vi "SpecAn_AMPM_ACP_TxP.vi"() -> ()   [LabVIEW 2016]
doc: "This example illustrates how to use the RFmx SpecAn and LTE personalities together with the RFSG drivers to perform ACP and EVM measurements with or without digital predistortion (DPD) of the waveform input to the DUT. \n\nDPD is a technique to optimize the operating point of power amplifiers and other non-linear RFIC devices. Power amplifiers are much more efficient if they operate near compression. However, compressing signal amplitudes can significantly deteriorate the amplified signal's quality both, in-band (e.g., EVM increases due to non-linear distortion of the signal's I/Q constellation) and out-of-band (e.g., ACP or SEM test fails due to spectral regrowth). With DPD, the original waveform is first pre-distorted in a way that matches the non-linear effects of the RFIC device before being fed through the device. The resulting output is a much cleaner amplified and/or filtered version of the original waveform. \n\nDifferent DPD models can be used to trade off performance with computational ease, with the Lookup-Table (LUT) model the simplest and the Generalized Memory Polynomial Model (GMP) the most complex. With a LUT, the DPD algorithm achieves gain and phase linearization on average. If you want to correct for memory effects - i.e., an output sample not only depends on the current input but also previous input samples; you will notice that a specific input power value translates into a range of gain and phase values - you would use one of the memory polynomial models. For these models, several parameters such as polynomial order and memory depth are available to fine-tune the model to the DUT behavior."
uses:
  Source/SG/Typedefs/LO Configruation.ctl
  <instrlib>/niRFSG/niRFSG.llb/niRFSG Exported Signal Destinations.ctl
  Source/SG/Typedefs/Instrument Configuration.ctl
  <instrlib>/niRFSG/niRFSG.llb/niRFSG Ref Clock Sources.ctl
  Source/SA/RFmxSpecAn/Typedefs/AMPM Configuration.ctl
  Source/SA/RFmxSpecAn/Typedefs/SpecAn Common Configuration.ctl
  Source/SA/RFmxSpecAn/Typedefs/ACP Common Configuration.ctl
  Source/SA/RFmxSpecAn/Typedefs/ACP Carrier Channel Configuration.ctl
  Source/SA/RFmxNR/Typedefs/NR ACP Offset Results.ctl
  Source/SA/RFmxSpecAn/Typedefs/ACP Offset Channel Configuration.ctl
  Source/SA/RFmxSpecAn/Typedefs/TxP Configuration.ctl
  <vilib>/RFmx/SpecAn/mx/RFmxSpecAn.llb/RFmxSpecAn Select Measurement (Single).vi
  Source/SG/SG.lvlib
  Source/SA/RFmxSpecAn/RFmxSpecAn.lvlib
  Source/SA/RFmxInstr/RFmxInstr.lvlib
  Source/SA/RFmxNR/RFmxNR.lvlib
panel:
  in  "Center Frequency / SG IF (Hz)":dbl=3500000000.0 format="%.6p"
  in  "Error Tab Control":enum32{"Page 1", "Page 2"}(tab)
  out "error out":errorcluster
  in  "Display Tab Control":enum32{"AMPM Results", "ACP Results", "TxP"}(tab)
  out "AM to AM Plot":T1(graph)
  out "AM to PM Plot":T2(graph)
  out "AMPM Measurement Results":T3 {"1 dB Compression Point (dBm)" format="%.2f"; "AM to PM Residual (deg)" format="%.2f"; "AM to AM Residual (dB)" format="%.2f"; "Mean RMS EVM (%)" format="%.2f"; "Mean Linear Gain (dB)" format="%.2f"}
  out "Spectrum":cluster{"x0":dbl, "dx":dbl, "y":sgl[]}(graph) caption="DUT Output Spectrum"
  out "Offset Results":T4[](array[typedef])
  out "Component Carrier Results":T5(array[cluster])
  out "Power Trace":cluster{"x0":dbl, "dx":dbl, "y":sgl[]}(graph)
  out "TxP Results":T6 {"Minimum Power (dBm)" format="%.2f"; "Maximum Power (dBm)" format="%.2f"; "Peak to Average Ratio (dB)" format="%.2f"; "Average Mean Power (dBm)" format="%.2f"}
  in  "Measurement Settings Tab Control":T7(tab)
  in  "TxP Config":T8={"Measurement Interval (s)"=0.001, "RBW"={"RBW Filter Type"=5, "RBW (Hz)"=20000000.0, "RRC Alpha"=0.01}, "VBW"={"VBW Auto"=1, "VBW (Hz)"=30000.0, "VBW to RBW Ratio"=3.0}, "Threshold"={"Threshold Enabled"=0, "Threshold Type"=0, "Threshold Level (dB or dBm)"=-20.0}, "Averaging"={"Averaging Count"=10, "Averaging Enabled"=0, "Averaging Type"=0}} {"Averaging"."Averaging Type" items=["RMS", "Log", "Scalar", "Max", "Min"]; "Averaging"."Averaging Enabled" items=["False", "True"]; "Threshold"."Threshold Level (dB or dBm)" format="%.2g"; "Threshold"."Threshold Type" items=["Relative", "Absolute"]; "Threshold"."Threshold Enabled" items=["False", "True"]; "VBW"."VBW to RBW Ratio" format="%#.6f"; "VBW"."VBW (Hz)" format="%.3p"; "VBW"."VBW Auto" items=["False", "True"]; "RBW"."RRC Alpha" format="%.3g"; "RBW"."RBW (Hz)" format="%.3p"; "RBW"."RBW Filter Type" items=["None"=5, "Gaussian"=1, "Flat"=2, "RRC"=6]; "Measurement Interval (s)" format="%.2p"}
  in  "RFmx SpecAn AMPM Configuration":T9={"Measurement Interval (s)"=0.0001, "DUT Average Input Power (dBm)"=-20.0, "Reference Waveform"={"x0"=0.0, "dx"=0.0, "y"=[]}, "Idle Duration Present"=0, "Signal Type"=0} {"Signal Type" items=["Modulated", "Tones"]; "Idle Duration Present" items=["False", "True"]; "Reference Waveform"."y" format="%.2f"; "Reference Waveform"."dx" format="%^.2e"; "Reference Waveform"."x0" format="%^.2e"; "DUT Average Input Power (dBm)" format="%.2f"; "Measurement Interval (s)" format="%.2p"}
  in  "ACP Common Configuration":T10={"Averaging Count"=10, "Averaging Enabled"=0, "Averaging Type"=0, "FFT Padding"=1.0, "FFT Window"=1, "Sweep Time Interval (s)"=0.001, "Sweep Time Auto"=1, "RBW Filter Type"=1, "RBW (Hz)"=10000.0, "RBW Auto"=1, "Power Units"=0} {"Power Units" items=["dBm", "dBm/Hz"]; "RBW Auto" items=["False", "True"]; "RBW (Hz)" format="%.3p"; "RBW Filter Type" items=["FFT Based", "Gaussian", "Flat", "Synch Tuned - 4", "Synch Tuned - 5"]; "Sweep Time Auto" items=["False", "True"]; "Sweep Time Interval (s)" format="%.2p"; "FFT Window" items=["None", "Flat Top", "Hanning", "Hamming", "Gaussian", "Blackman", "Blackman-Harris", "Kaiser-Bessel"]; "FFT Padding" format="%.2f"; "Averaging Type" items=["RMS", "Log", "Scalar", "Max", "Min", "Vector"]; "Averaging Enabled" items=["False", "True"]}
  in  "ACP Carrier Channel Configuration":T11=[{"Carrier Frequency (Hz)"=0.0, "Integration Bandwidth (Hz)"=18000000.0, "RRC Filter"={"Alpha"=0.22, "Enabled"=0}, "Mode"=1}] {"Mode" items=["Passive", "Active"]; "Carrier Frequency (Hz)" format="%.3p"; "RRC Filter"."Enabled" items=["False", "True"]; "RRC Filter"."Alpha" format="%.3g"; "Integration Bandwidth (Hz)" format="%.3p"}
  in  "ACP Offset Channel Configuration":T12=[{"Offset Frequency"={"Frequency (Hz)"=20000000.0, "Sideband"=2}, "Offset Power Reference"={"Specific Index"=0, "Carrier"=0}, "Integration Bandwidth (Hz)"=18000000.0, "Relative Attenuation (dB)"=0.0, "RRC Filter"={"Alpha"=0.22, "Enabled"=0}, "Enabled"=1}, {"Offset Frequency"={"Frequency (Hz)"=12500000.0, "Sideband"=2}, "Offset Power Reference"={"Specific Index"=0, "Carrier"=0}, "Integration Bandwidth (Hz)"=3840000.0, "Relative Attenuation (dB)"=0.0, "RRC Filter"={"Alpha"=0.22, "Enabled"=0}, "Enabled"=1}, {"Offset Frequency"={"Frequency (Hz)"=17500000.0, "Sideband"=2}, "Offset Power Reference"={"Specific Index"=0, "Carrier"=0}, "Integration Bandwidth (Hz)"=3840000.0, "Relative Attenuation (dB)"=0.0, "RRC Filter"={"Alpha"=0.22, "Enabled"=0}, "Enabled"=1}] {"Enabled" items=["False", "True"]; "Offset Power Reference"."Carrier" items=["Closest", "Highest", "Composite", "Specific"]; "RRC Filter"."Enabled" items=["False", "True"]; "RRC Filter"."Alpha" format="%.3g"; "Relative Attenuation (dB)" format="%.2f"; "Integration Bandwidth (Hz)" format="%.3p"; "Offset Frequency"."Sideband" items=["Neg", "Pos", "Both"]; "Offset Frequency"."Frequency (Hz)" format="%.3p"}
  in  "Resource Control":enum32{"RFSG", "RFSA", "LO Config"}(tab)
  in  "Marker Event Output Terminal":T13="PXI_Trig0"
  in  "Reference Waveform File Path":path=path "C:/Users/Public/Documents/National Instruments/RFIC Test Software/Waveforms/LTE_FDD_UL_1x20MHz_256QAM_OS4.tdms"
  in  "RFSG Resource Name":refnum<k15>="RFSG"
  in  "SG Configuration":T14={"Reference Clock Source"="PXI_CLK", "Carrier Frequency (Hz)"=3500000000.0, "DUT Average Input Power (dBm)"=-10.0, "External Attenuation (dB)"=0.0, "SelectedPorts"=""} {"Carrier Frequency (Hz)" format="%#_6p"}
  in  "RFSA Resource Name":refnum<k15>="RFSA"
  in  "RFmx SpecAn Spectrum Configuration":T16={"Center Frequency (Hz)"=1000000000.0, "Reference Level (dBm)"=0.0, "External Attenuation (dB)"=0.0, "Digital Edge Source"="PXI_Trig0", "Digital Edge"=0, "Trigger Delay (s)"=0.0, "Enable Trigger?"=TRUE, "Frequency Reference Source"="PXI_Clk", "SelectedPorts"=""} {"Trigger Delay (s)" format="%.2p"; "Digital Edge" items=["Rising Edge", "Falling Edge"]; "External Attenuation (dB)" format="%.2f"; "Reference Level (dBm)" format="%.2f"; "Center Frequency (Hz)" format="%.6p"}
  in  "LO Configuration":T17={"LO Sharing Mode"=1, "LO Offset Mode"=1, "LO Offset (Hz)"=0.0} {"LO Offset Mode" items=["NoOffset", "Automatic", "User Defined"]; "LO Sharing Mode" items=["None", "Automatic", "Manual"]}
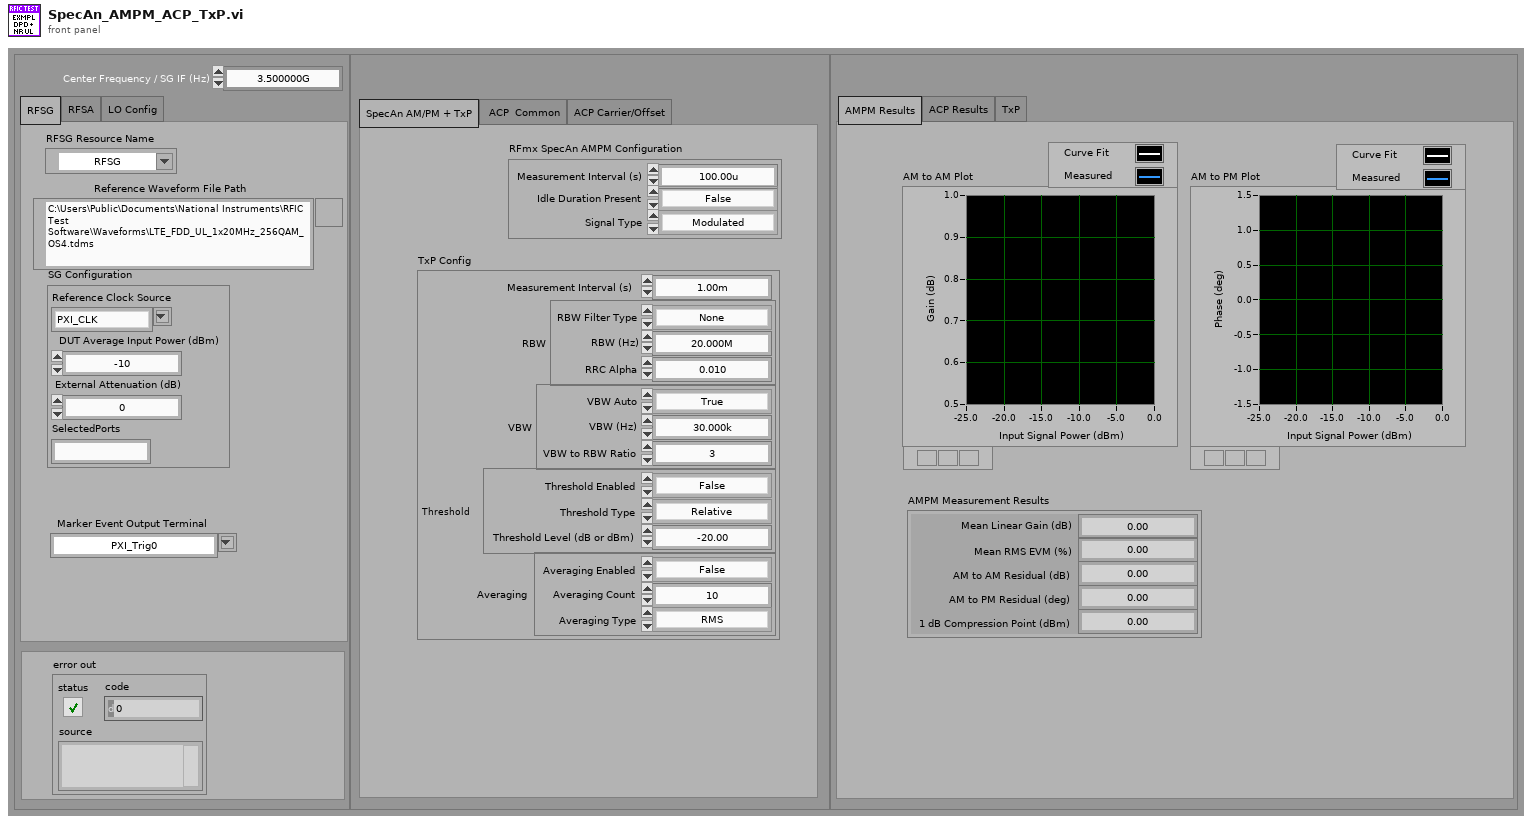
[diagram p1: front panel]
types:
  T1 = cluster{"Input Powers (dBm)":sgl[], "Curve Fit AM to AM (dB)":sgl[]}[]
  T2 = cluster{"Input Powers (dBm)":sgl[], "Curve Fit AM to PM (dB)":sgl[]}[]
  T3 = cluster{"Mean Linear Gain (dB)":dbl, "Mean RMS EVM (%)":dbl, "AM to AM Residual (dB)":dbl, "AM to PM Residual (deg)":dbl, "1 dB Compression Point (dBm)":dbl}
  T4 = typedef "RFmxNR.lvlib/NR ACP Offset Results.ctl" = cluster{"Upper Absolute Power (dBm)":dbl, "Lower Absolute Power (dBm)":dbl, "Lower Relative Power (dB)":dbl, "Upper Relative Power (dB)":dbl, "Offset Frequency (Hz)":dbl, "Offset Integration Bandwidth (Hz)":dbl}
  T5 = cluster{"Carrier Frequency (Hz)":dbl, "Integration Bandwidth (Hz)":dbl, "Absolute Power (dBm or dBm/Hz)":dbl, "Total Relative Power (dB)":dbl}[]
  T6 = cluster{"Average Mean Power (dBm)":dbl, "Peak to Average Ratio (dB)":dbl, "Maximum Power (dBm)":dbl, "Minimum Power (dBm)":dbl, "Power Trace":cluster{"x0":dbl, "dx":dbl, "y":sgl[]}}
  T7 = enum32{"SpecAn AM/PM + TxP", " ACP  Common", "ACP Carrier/Offset"}
  T8 = typedef "RFmxSpecAn.lvlib/TxP Configuration.ctl" = cluster{"Measurement Interval (s)":dbl, "RBW":cluster{"RBW Filter Type":i32, "RBW (Hz)":dbl, "RRC Alpha":dbl}, "VBW":cluster{"VBW Auto":i32, "VBW (Hz)":dbl, "VBW to RBW Ratio":dbl}, "Threshold":cluster{"Threshold Enabled":i32, "Threshold Type":i32, "Threshold Level (dB or dBm)":dbl}, "Averaging":cluster{"Averaging Count":i32, "Averaging Enabled":i32, "Averaging Type":i32}}
  T9 = typedef "RFmxSpecAn.lvlib/AMPM Configuration.ctl" = cluster{"Measurement Interval (s)":dbl, "DUT Average Input Power (dBm)":dbl, "Reference Waveform":cluster{"x0":dbl, "dx":dbl, "y":csg[]}, "Idle Duration Present":i32, "Signal Type":i32}
  T10 = typedef "RFmxSpecAn.lvlib/ACP Common Configuration.ctl" = cluster{"Averaging Count":i32, "Averaging Enabled":i32, "Averaging Type":i32, "FFT Padding":dbl, "FFT Window":i32, "Sweep Time Interval (s)":dbl, "Sweep Time Auto":i32, "RBW Filter Type":i32, "RBW (Hz)":dbl, "RBW Auto":i32, "Power Units":i32}
  T11 = typedef "RFmxSpecAn.lvlib/ACP Carrier Channel Configuration.ctl" = cluster{"Carrier Frequency (Hz)":dbl, "Integration Bandwidth (Hz)":dbl, "RRC Filter":cluster{"Alpha":dbl, "Enabled":i32}, "Mode":i32}[]
  T12 = typedef "RFmxSpecAn.lvlib/ACP Offset Channel Configuration.ctl" = cluster{"Offset Frequency":cluster{"Frequency (Hz)":dbl, "Sideband":i32}, "Offset Power Reference":cluster{"Specific Index":i32, "Carrier":i32}, "Integration Bandwidth (Hz)":dbl, "Relative Attenuation (dB)":dbl, "RRC Filter":cluster{"Alpha":dbl, "Enabled":i32}, "Enabled":i32}[]
  T13 = typedef "niRFSG Exported Signal Destinations.ctl" = string
  T14 = typedef "SG.lvlib/Instrument Configuration.ctl" = cluster{"Reference Clock Source":T15, "Carrier Frequency (Hz)":dbl, "DUT Average Input Power (dBm)":dbl, "External Attenuation (dB)":dbl, "SelectedPorts":string}
  T15 = typedef "niRFSG Ref Clock Sources.ctl" = string
  T16 = typedef "RFmxSpecAn.lvlib/SpecAn Common Configuration.ctl" = cluster{"Center Frequency (Hz)":dbl, "Reference Level (dBm)":dbl, "External Attenuation (dB)":dbl, "Digital Edge Source":string, "Digital Edge":i32, "Trigger Delay (s)":dbl, "Enable Trigger?":bool, "Frequency Reference Source":string, "SelectedPorts":string}
  T17 = typedef "SG.lvlib/LO Configruation.ctl" = cluster{"LO Sharing Mode":i32, "LO Offset Mode":i32, "LO Offset (Hz)":dbl}
  T18 = enum16{"ACP", "CCDF", "CHP", "FCnt", "Harmonics", "OBW", "SEM", "Spectrum", "Spur", "TXP", "AMPM", "DPD", "IQ", "IM", "NF", "PhaseNoise"}
  T19 = typedef "SG.lvlib/Waveform.ctl" = cluster{"Waveform Name":string, "Waveform":cluster{"x0":dbl, "dx":dbl, "y":csg[]}, "Signal Bandwidth (Hz)":dbl, "PAPR (dB)":dbl, "Burst Length (s)":dbl, "Sample Rate":dbl, "Burst Start Locations":i32[], "Burst Stop Locations":i32[], "Idle Duration Present?":bool, "Runtime Scaling":dbl}
  T20 = typedef "RFmxSpecAn.lvlib/AMPM Results.ctl" = cluster{"Mean Linear Gain (dB)":dbl, "1 dB Compression Point (dBm)":dbl, "Mean RMS EVM (%)":dbl, "AM to AM Residual (dB)":dbl, "AM to PM Residual (deg)":dbl, "AMAM vs Pin":cluster{"Input Powers (dBm)":sgl[], "Measured AM to AM (dB)":sgl[]}, "AMAM Curve Fit vs Pin":cluster{"Input Powers (dBm)":sgl[], "Curve Fit AM to AM (dB)":sgl[]}, "AMPM vs Pin":cluster{"Input Powers (dBm)":sgl[], "Measured AM to PM (dB)":sgl[]}, "AMPM Curve Fit vs Pin":cluster{"Input Powers (dBm)":sgl[], "Curve Fit AM to PM (dB)":sgl[]}}
  T21 = cluster{"Input Powers (dBm)":sgl[], "Curve Fit AM to AM (dB)":sgl[]}
  T22 = cluster{"Input Powers (dBm)":sgl[], "Measured AM to AM (dB)":sgl[]}
  T23 = cluster{"Input Powers (dBm)":sgl[], "Curve Fit AM to PM (dB)":sgl[]}
  T24 = cluster{"Input Powers (dBm)":sgl[], "Measured AM to PM (dB)":sgl[]}
  T25 = cluster{"Input Powers (dBm)":sgl[], "Measured AM to PM (dB)":sgl[]}[]
  T26 = cluster{"Input Powers (dBm)":sgl[], "Measured AM to AM (dB)":sgl[]}[]
  T27 = typedef "RFmxSpecAn.lvlib/ACP Results.ctl" = cluster{"Offset Results":T4[], "Component Carrier Results":cluster{"Carrier Frequency (Hz)":dbl, "Integration Bandwidth (Hz)":dbl, "Absolute Power (dBm or dBm/Hz)":dbl, "Total Relative Power (dB)":dbl}[], "Spectrum (dBm or dBm/Hz)":cluster{"x0":dbl, "dx":dbl, "y":sgl[]}, "Total Carrier Power (dBm or dBm/Hz)":dbl}
  T28 = typedef "RFmxSpecAn.lvlib/TxP Results.ctl" = cluster{"Average Mean Power (dBm)":dbl, "Peak to Average Ratio (dB)":dbl, "Maximum Power (dBm)":dbl, "Minimum Power (dBm)":dbl, "Power Trace":cluster{"x0":dbl, "dx":dbl, "y":sgl[]}}
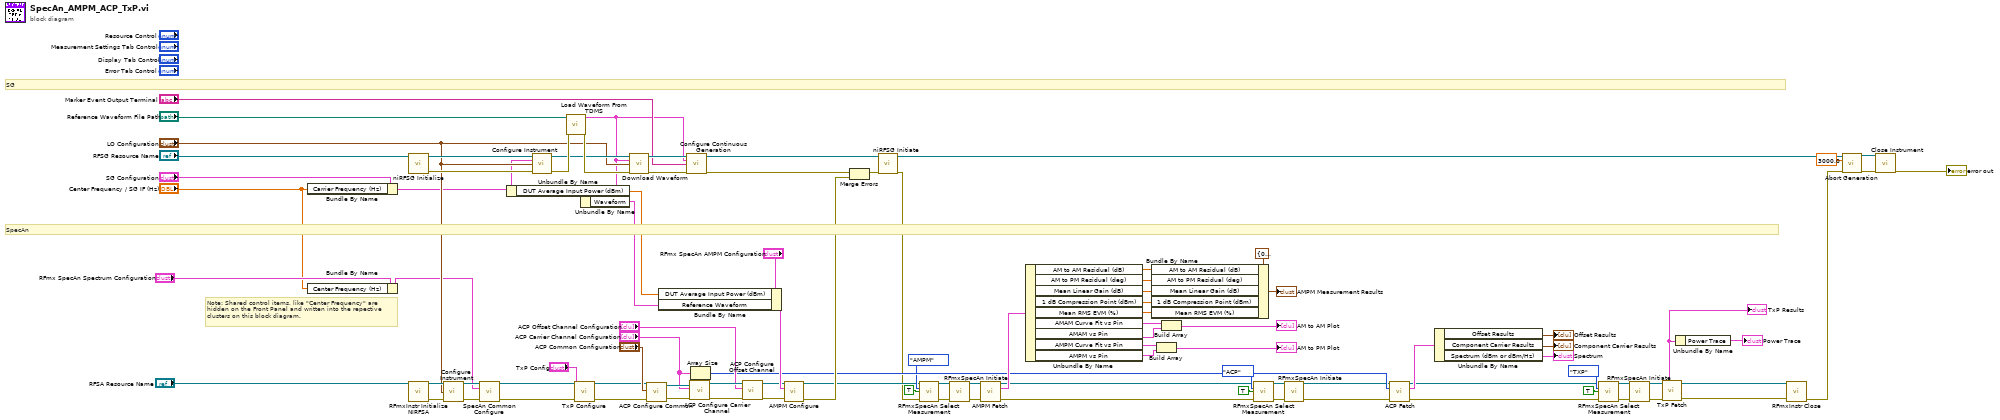
[diagram p0: block diagram]
diagram:
  # "Note: Shared control items, like \"Center Frequency\" are \nhidden on the Front Panel and written into the repective \nclusters on this block diagram."
  # "SG"
  # "SpecAn"
  n1 = Bundle By Name(cluster="SG Configuration", "Carrier Frequency (Hz)"="Center Frequency / SG IF (Hz)") -> (w69:T14)
  n2 = Bundle By Name(cluster="RFmx SpecAn Spectrum Configuration", "Center Frequency (Hz)"="Center Frequency / SG IF (Hz)") -> (w36:T16)
  n3 = call <instrlib>:"niRFSG Initialize.vi"("resource name"="RFSG Resource Name") -> ("instrument handle"=w90:refnum<k15>, "error out"=w89:errorcluster)  [unwired: 13 in]
  n4 = call <vilib>:"RFmxInstr Initialize NIRFSA.vi"("Resource Name"="RFSA Resource Name") -> ("Instrument Handle Out"=w78:refnum<k21>, "error out"=w76:errorcluster)  [unwired: 12 in, 1 out]
  n5 = call "Configure Instrument.vi"("RFmx Handle In"=w78, "LO Configuration"="LO Configuration", "error in (no error)"=w76) -> ("RFmx Handle Out"=w77:refnum<k21>, "error out"=w74:errorcluster)  [unwired: 11 in]
  n6 = call "SpecAn Common Configure.vi"("RFmx Handle In"=w77, "RFmx SpecAn Spectrum Configuration"=w36, "error in (no error)"=w74) -> ("RFmx Handle Out"=w34:refnum<k21>, "error out"=w32:errorcluster)  [unwired: 11 in]
  n7 = Unbundle By Name(w69) -> ("DUT Average Input Power (dBm)"=w68:dbl)
  n8 = call "Configure Instrument.vi"("RFSG Session In"=w90, "SG Configuration"=w69, "LO Configuration"="LO Configuration", "error in (no error)"=w89) -> ("RFSG Session Out"=w95:refnum<k15>, "error out"=w97:errorcluster)  [unwired: 10 in]
  n9 = call "Load Waveform From TDMS.vi"("TDMS File Path"="Reference Waveform File Path", "error in (no error)"=w97) -> ("Waveform"=w67:T19, "error out"=w96:errorcluster)  [unwired: 12 in]
  n10 = call "TxP Configure.vi"("Instrument Handle In"=w34, "TxP Config"="TxP Config", "error in (no error)"=w32) -> ("Instrument Handle Out"=w33:refnum<k21>, "error out"=w31:errorcluster)  [unwired: 11 in]
  n11 = Unbundle By Name(w67) -> ("Waveform"=w66:cluster{"x0":dbl, "dx":dbl, "y":csg[]})
  n12 = call "Download Waveform.vi"("RFSG handle"=w95, "Waveform In"=w67, "LO Configuration"="LO Configuration", "error in (no error)"=w96) -> ("RFSG handle out"=w88:refnum<k15>, "error out"=w86:errorcluster)  [unwired: 10 in]
  n13 = call "ACP Configure Common.vi"("error in (no error)"=w31, "ACP Common Configuration"="ACP Common Configuration", "Instrument Handle In"=w33) -> ("error out"=w48:errorcluster, "Instrument Handle Out"=w49:refnum<k21>)  [unwired: 7 in]
  n14 = Bundle By Name(cluster="RFmx SpecAn AMPM Configuration", "DUT Average Input Power (dBm)"=w68, "Reference Waveform"=w66) -> (w70:T9)
  n15 = call "Configure Continuous Generation.vi"("RFSG handle"=w88, "Waveform"=w67, "Waveform Start Trigger Export"="Marker Event Output Terminal", "error in"=w86) -> ("RFSG handle out"=w87:refnum<k15>, "error out"=w85:errorcluster)  [unwired: 10 in]
  n16 = call "ACP Configure Carrier Channel.vi"("error in (no error)"=w48, "ACP Carrier Channel Configuration"="ACP Carrier Channel Configuration", "Instrument Handle In"=w49) -> ("error out"=w46:errorcluster, "Instrument Handle Out"=w47:refnum<k21>)  [unwired: 7 in]
  n17 = Array Size(array="ACP Carrier Channel Configuration") -> (size(s)=w38:i32)
  n18 = call "ACP Configure Offset Channel.vi"("error in (no error)"=w46, "ACP Offset Channel Configuration"="ACP Offset Channel Configuration", "Instrument Handle In"=w47) -> ("error out"=w45:errorcluster, "Instrument Handle Out"=w41:refnum<k21>)  [unwired: 7 in]
  n19 = call "AMPM Configure.vi"("RFmx Handle In"=w41, "RFmx SpecAn AMPM Configuration"=w70, "error in (no error)"=w45) -> ("RFmx Handle Out"=w16:refnum<k21>, "error out"=w72:errorcluster)  [unwired: 11 in]
  n20 = Merge Errors(w85, w72) -> (w84:errorcluster)
  n21 = call <instrlib>:"niRFSG Initiate.vi"("instrument handle"=w87, "error in"=w84) -> ("instrument handle out"=w94:refnum<k15>, "error out"=w15:errorcluster)  [unwired: 12 in]
  n22 = call-poly <vilib>:"RFmxSpecAn Select Measurement.vi"("Instrument Handle In"=w16, "Measurement"=T18."AMPM", "Enable All Traces"=TRUE, "error in (no error)"=w15) -> ("Instrument Handle Out"=w25:refnum<k21>, "error out"=w26:errorcluster)  [unwired: 10 in]
  n23 = call <vilib>:"RFmxSpecAn Initiate.vi"("Instrument Handle In"=w25, "error in (no error)"=w26) -> ("Instrument Handle Out"=w11:refnum<k21>, "error out"=w14:errorcluster)  [unwired: 11 in, 1 out]
  n24 = call "AMPM Fetch.vi"("RFmx Handle In"=w11, "error in (no error)"=w14) -> ("RFmx Handle Out"=w10:refnum<k21>, "AMPM Results"=w64:T20, "error out"=w13:errorcluster)  [unwired: 11 in]
  n25 = Unbundle By Name(w64) -> ("AM to AM Residual (dB)"=w63:dbl, "AM to PM Residual (deg)"=w62:dbl, "Mean Linear Gain (dB)"=w60:dbl, "1 dB Compression Point (dBm)"=w59:dbl, "Mean RMS EVM (%)"=w58:dbl, "AMAM Curve Fit vs Pin"=w57:T21, "AMAM vs Pin"=w56:T22, "AMPM Curve Fit vs Pin"=w54:T23, "AMPM vs Pin"=w53:T24)
  n26 = Bundle By Name(cluster=T3 {"Mean Linear Gain (dB)"=0.0, "Mean RMS EVM (%)"=0.0, "AM to AM Residual (dB)"=0.0, "AM to PM Residual (deg)"=0.0, "1 dB Compression Point (dBm)"=0.0} ("Measurement"), "AM to AM Residual (dB)"=w63, "AM to PM Residual (deg)"=w62, "Mean Linear Gain (dB)"=w60, "1 dB Compression Point (dBm)"=w59, "Mean RMS EVM (%)"=w58) -> (→"AMPM Measurement Results":T3)
  n27 = Build Array(w54, w53) -> (→"AM to PM Plot":T25)
  n28 = Build Array(w57, w56) -> (→"AM to AM Plot":T26)
  n29 = call-poly <vilib>:"RFmxSpecAn Select Measurement.vi"("Instrument Handle In"=w10, "Measurement"=T18."ACP", "Enable All Traces"=TRUE, "error in (no error)"=w13) -> ("Instrument Handle Out"=w21:refnum<k21>, "error out"=w22:errorcluster)  [unwired: 10 in]
  n30 = call <vilib>:"RFmxSpecAn Initiate.vi"("Instrument Handle In"=w21, "error in (no error)"=w22) -> ("Instrument Handle Out"=w9:refnum<k21>, "error out"=w12:errorcluster)  [unwired: 11 in, 1 out]
  n31 = call "ACP Fetch.vi"("RFmx Handle In"=w9, "Num Carrier Channels"=w38, "error in (no error)"=w12) -> ("RFmx Handle Out"=w8:refnum<k21>, "ACP Results"=w44:T27, "error out"=w7:errorcluster)  [unwired: 10 in]
  n32 = Unbundle By Name(w44) -> ("Offset Results"=→"Offset Results":T4[], "Component Carrier Results"=→"Component Carrier Results":T5, "Spectrum (dBm or dBm/Hz)"=→"Spectrum":cluster{"x0":dbl, "dx":dbl, "y":sgl[]})
  n33 = call-poly <vilib>:"RFmxSpecAn Select Measurement.vi"("Instrument Handle In"=w8, "Measurement"=T18."TXP", "Enable All Traces"=TRUE, "error in (no error)"=w7) -> ("Instrument Handle Out"=w17:refnum<k21>, "error out"=w18:errorcluster)  [unwired: 10 in]
  n34 = call <vilib>:"RFmxSpecAn Initiate.vi"("Instrument Handle In"=w17, "error in (no error)"=w18) -> ("Instrument Handle Out"=w6:refnum<k21>, "error out"=w3:errorcluster)  [unwired: 11 in, 1 out]
  n35 = call "TxP Fetch.vi"("error in (no error)"=w3, "Instrument Handle In"=w6) -> ("error out"=w2:errorcluster, "TxP Results"=w5:T28, "Instrument Handle Out"=w30:refnum<k21>)  [unwired: 7 in]
  "TxP Results" <- w5
  n36 = Unbundle By Name(w5) -> ("Power Trace"=→"Power Trace":cluster{"x0":dbl, "dx":dbl, "y":sgl[]})
  n37 = call <vilib>:"RFmxInstr Close.vi"("Instrument Handle In"=w30, "error in (no error)"=w2) -> ("error out"=w73:errorcluster)  [unwired: 13 in]
  n38 = call "Abort Generation.vi"("RFSG handle"=w94, "Timeout (ms)"=3000.0, "error in (no error)"=w73) -> ("RFSG handle out"=w93:refnum<k15>, "error out"=w92:errorcluster)  [unwired: 11 in]
  n39 = call "Close Instrument.vi"("RFSG Handle"=w93, "error in (no error)"=w92) -> ("error out"=→"error out":errorcluster)  [unwired: 13 in]
